vi "Test.vi"() -> ()   [LabVIEW 2016]
uses:
  src/Log4Lv/Operate/PrintError.vi
  src/Log4Lv/Operate/Info.vi
  src/Log4Lv/Operate/Error.vi
  src/Log4Lv/Operate/Debug.vi
  src/Log4Lv/Operate/Warn.vi
  src/Log4Lv/Log4Lv.lvlib
panel:
  in  "Log Config File":string=".\\Log4Lv.ini"
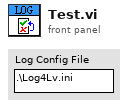
[diagram p1: front panel]
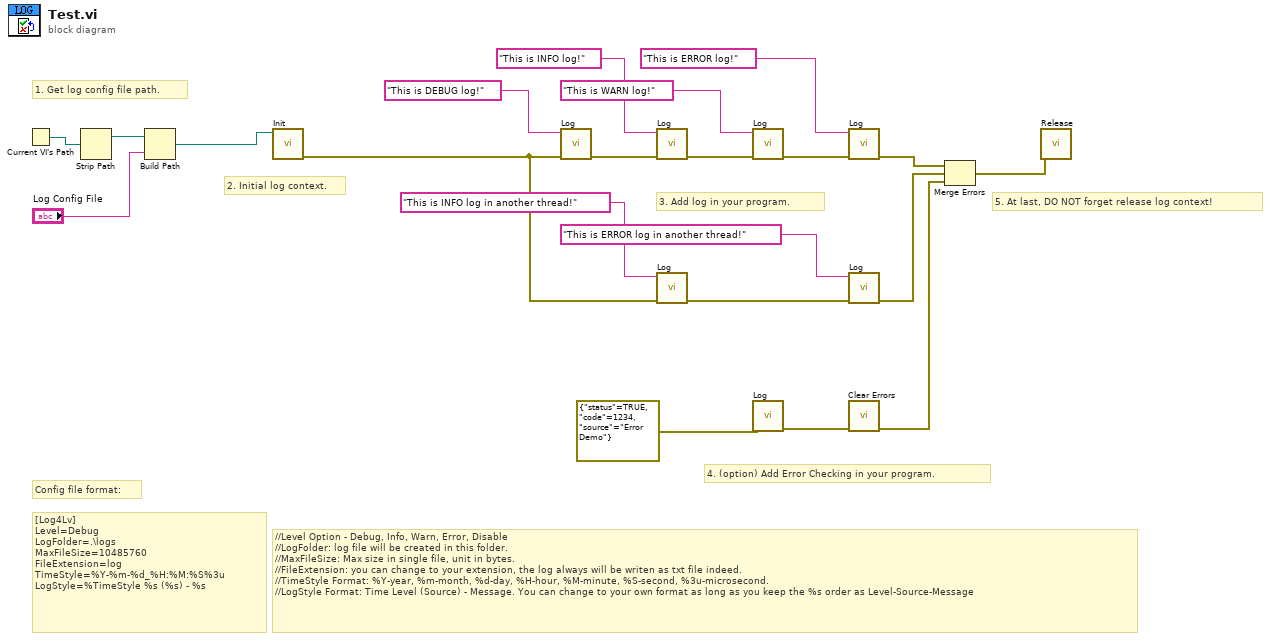
[diagram p0: block diagram]
diagram:
  # "//Level Option - Debug, Info, Warn, Error, Disable\n//LogFolder: log file will be created in this folder.\n//MaxFileSize: Max size in single file, unit in bytes.\n//FileExtension: you can change to your extension, the log always will be writen as txt file indeed.\n//TimeStyle Format: %Y-year, %m-month, %d-day, %H-hour, %M-minute, %S-second, %3u-microsecond.\n//LogStyle Format: Time Level (Source) - Message. You can change to your own format as long as you keep the %s order as Level-Source-Message"
  # "[Log4Lv]\nLevel=Debug\nLogFolder=.\\logs\nMaxFileSize=10485760\nFileExtension=log\nTimeStyle=%Y-%m-%d_%H:%M:%S%3u\nLogStyle=%TimeStyle %s (%s) - %s"
  # "Config file format:"
  # "5. At last, DO NOT forget release log context!"
  # "4. (option) Add Error Checking in your program."
  # "3. Add log in your program."
  # "2. Initial log context."
  # "1. Get log config file path."
  n1 = Current VI's Path() -> (path=w15:path)
  n2 = Strip Path(path=w15) -> (stripped path=w14:path)  [unwired: 1 out]
  n3 = Build Path(base path=w14, name or relative path="Log Config File") -> (appended path=w12:path)
  n4 = call "Init.vi"("Config File"=w12) -> ("error out"=w4:errorcluster)  [unwired: 10 in]
  n5 = call-poly "Log.vi"("error in (no error)"=w4, "Message"="This is DEBUG log!") -> ("error out"=w20:errorcluster)  [unwired: 9 in]
  n6 = call-poly "Log.vi"("error in (no error)"=w20, "Message"="This is INFO log!") -> ("error out"=w21:errorcluster)  [unwired: 9 in]
  n7 = call-poly "Log.vi"("error in (no error)"=w4, "Message"="This is INFO log in another thread!") -> ("error out"=w8:errorcluster)  [unwired: 9 in]
  n8 = call-poly "Log.vi"("error in (no error)"=w21, "Message"="This is WARN log!") -> ("error out"=w11:errorcluster)  [unwired: 9 in]
  n9 = call-poly "Log.vi"("error in (no error)"=errorcluster {"status"=TRUE, "code"=1234, "source"="Error Demo"} ("error constant")) -> ("error out"=w2:errorcluster)  [unwired: 10 in]
  n10 = call-poly "Log.vi"("error in (no error)"=w11, "Message"="This is ERROR log!") -> ("error out"=w6:errorcluster)  [unwired: 9 in]
  n11 = call-poly "Log.vi"("error in (no error)"=w8, "Message"="This is ERROR log in another thread!") -> ("error out"=w5:errorcluster)  [unwired: 9 in]
  n12 = call <vilib>:"Clear Errors.vi"("error in (no error)"=w2) -> ("error out"=w1:errorcluster)  [unwired: 5 in, 1 out]
  n13 = Merge Errors(w6, w5, w1) -> (w19:errorcluster)
  n14 = call "Release.vi"("error in (no error)"=w19) -> ()  [unwired: 10 in, 1 out]
